vi "tdms viewer.vi"() -> ()   [LabVIEW 2022 SP3]
uses:
  <vilib>/Utility/TDMS File Viewer/NI_TDMS File Viewer.lvlib
panel:
  in  "file in":path
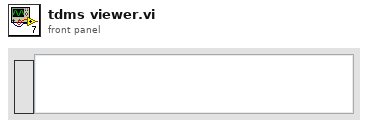
[diagram p1: front panel]
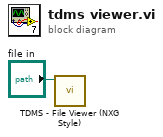
[diagram p0: block diagram]
diagram:
  n1 = call <vilib>:"TDMS - File Viewer (NXG Style).vi"("file in"="file in") -> ()  [unwired: 9 in, 2 out]
